vi "Get Instrument.vi"(8 "error in (no error)":errorcluster caption="entrée d'erreur (pas d'erreur)", 11 "Class Event (Default) en entrée":refnum<class "Class Event (Default).lvclass">) -> (0 "error out":errorcluster caption="sortie d'erreur", 2 "Library Instruments.lvlib:Class Instrument (Default).lvclass":refnum<class "Class Instrument (Default).lvclass">, 3 "Class Event (Default) en sortie":refnum<class "Class Event (Default).lvclass">)   [LabVIEW 2020, in "Library Instrument & Equipement.lvlib" / "Library Event.lvlib" / "Class Event (Default).lvclass"]
uses:
  Class Event (Default).lvclass
  Instrument/Instrument (Default)/Class Instrument (Default).lvclass
  Class Event (Default).lvclass/Class Event (Default).ctl
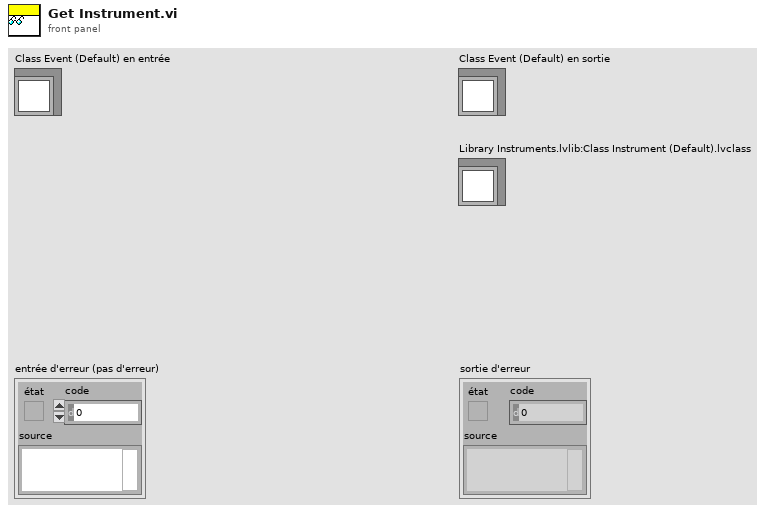
[diagram p1: front panel]
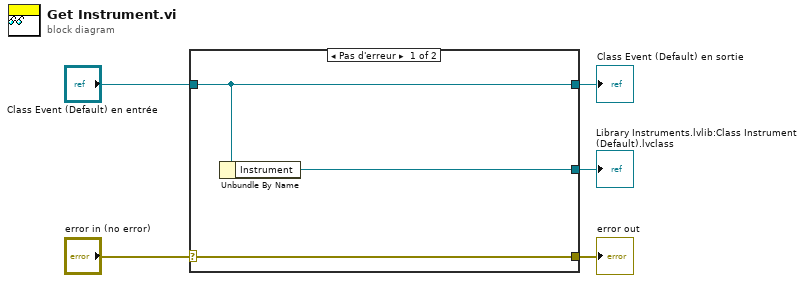
[diagram p0: block diagram]
diagram:
  n1 = case shown="Pas d'erreur" "error in (no error)" {
    selector: "error in (no error)" -> [w8 w9]
    tunnel: [w8 w9] -> w4
    tunnel: [w7 w10] -> w2
    tunnel: "Class Event (Default) en entrée" -> [w7 w10]
    tunnel: [w6 _] -> w1
    frame No Error {
      n2 = Unbundle By Name(w7) -> ("Instrument"=w6:refnum<class "Class Instrument (Default).lvclass">)
    }
    frame Error {
    }
  }
  "error out" <- w4
  "Class Event (Default) en sortie" <- w2
  "Library Instruments.lvlib:Class Instrument (Default).lvclass" <- w1
